vi "DataLog Read Index File.vi"(0 "tag log directory":path, 11 "error in (no error)":errorcluster) -> (4 "dup tag log directory":path, 8 "chunk start timestamps":dbl[](array[numeric]) format="%<%I:%M:%S %p\n%m/%d/%Y>T", 10 "write index":dbl, 15 "error out":errorcluster)   [LabVIEW 2012]
doc: "Read the indices from file including as well as the chunk start timestamps. These are the timestamps of first point of the subsequent chunks. Via these timestamps it is possible to quickly locate the chunk containing a particular time range."
uses:
  glb_DataLog MCVD.vi
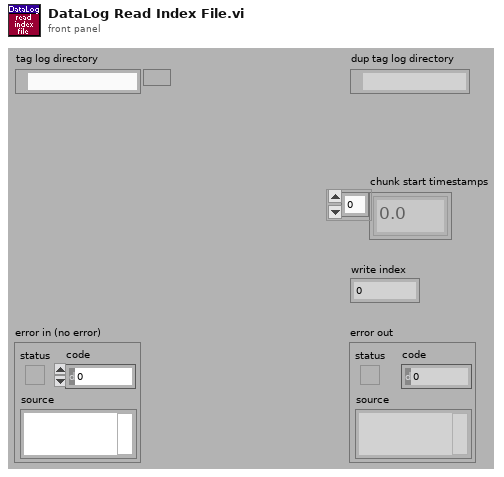
[diagram p1: front panel]
types:
  T1 = enum16{"read/write", "read-only", "write-only", "write-only (truncate)"}
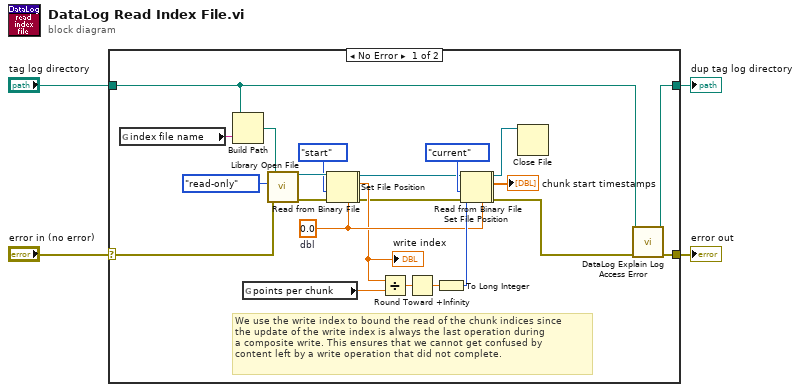
[diagram p0: block diagram]
diagram:
  n1 = case shown="No Error" "error in (no error)" {
    selector: "error in (no error)" -> [w29 w32]
    tunnel: [w12 w32] -> w4
    tunnel: "tag log directory" -> [w10 w31]
    tunnel: [w9 w31] -> w1
    frame No Error {
      w16 = 0.0  # dbl
      # "We use the write index to bound the read of the chunk indices since\nthe update of the write index is always the last operation during\na composite write. This ensures that we cannot get confused by\ncontent left by a write operation that did not complete."
      n2 = global read "glb_DataLog MCVD.vi" "index file name"() -> (w30:string)
      n3 = Build Path(base path=w10, name or relative path=w30) -> (appended path=w27:path)
      n4 = global read "glb_DataLog MCVD.vi" "points per chunk"() -> (w22:dbl)
      n5 = call "Library Open File.vi"("error in (no error)"=w29, "open mode (read/write)"=T1."read-only" ("open mode (0)"), "file path"=w27) -> ("error out"=w26:errorcluster, "refnum"=w25:refnum<file>)  [unwired: 3 in]
      n6 = Set File Position(refnum=w25, from (0:start)=enum16{"start", "end", "current"}."start" ("pos mode (0:2)"), error in=w26) -> (refnum out=w6:refnum<file>, error out=w5:errorcluster)  [unwired: 1 in]
      n7 = Read from Binary File(5:w16, 8:w5, 11:w6) -> (0:w13:errorcluster, 2:w15:dbl, 3:w14:refnum<file>)  [unwired: 3 in, 1 out]
      "write index" <- w15
      n8 = Divide(x=w15, y=w22) -> (x/y=w21:dbl)
      n9 = Round Toward +Infinity(x=w21) -> (ceil(x): smallest int >= x=w20:dbl)
      n10 = To Long Integer(number=w20) -> (32bit integer=w19:i32)
      n11 = Set File Position(refnum=w14, from (0:start)=enum16{"start", "end", "current"}."current" ("pos mode (0:2)"), error in=w13) -> (refnum out=w8:refnum<file>, error out=w7:errorcluster)  [unwired: 1 in]
      n12 = Read from Binary File(5:w16, 8:w7, 10:w19, 11:w8) -> (0:w11:errorcluster, 2:→"chunk start timestamps":dbl[], 3:w23:refnum<file>)  [unwired: 2 in, 1 out]
      n13 = Close File(refnum=w23) -> ()  [unwired: 1 in, 2 out]
      n14 = call "DataLog Explain Log Access Error.vi"("tag log directory"=w10, "error in"=w11) -> ("dup tag log directory"=w9:path, "error out"=w12:errorcluster)  [unwired: 12 in]
    }
    frame Error {
    }
  }
  "error out" <- w4
  "dup tag log directory" <- w1
